vi "ui get all file type duplicate list.vi"() -> ()   [LabVIEW 2023]
panel:
  out "duplicates file count":i32
  in  "Root folder path of all files":path
  out "Destination":path[](array[path])
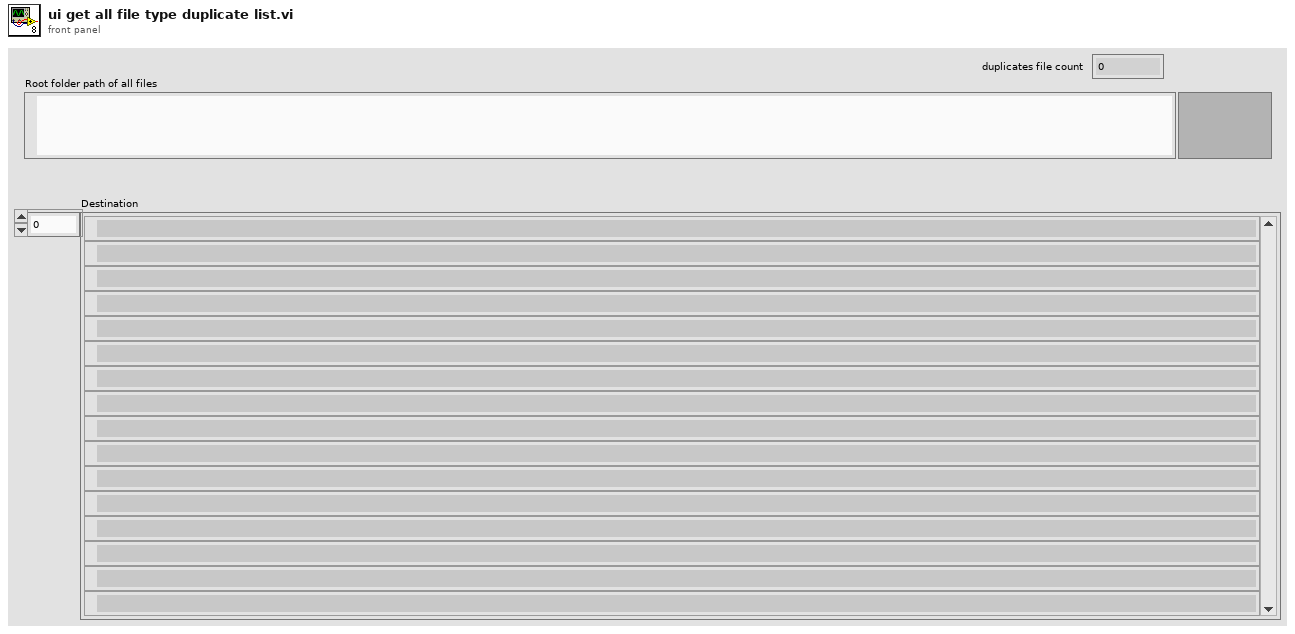
[diagram p1: front panel]
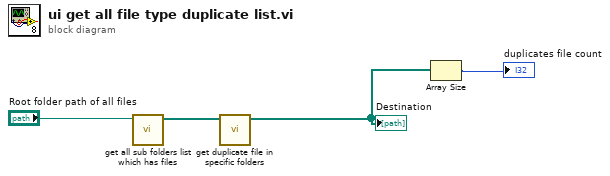
[diagram p0: block diagram]
diagram:
  n1 = call "get all sub folders list which has files.vi"("Folder Path"="Root folder path of all files") -> ("All Folders"=w2:path[])  [unwired: 10 in]
  n2 = call "get duplicate file in specific folders.vi"("All Folders"=w2) -> ("Array"=w1:path[])  [unwired: 10 in]
  "Destination" <- w1
  n3 = Array Size(array=w1) -> (size(s)=→"duplicates file count":i32)
